vi "String_Conversion_OP110.vi"(11 "String in":string) -> (2 "Array":string[](array[string]), 3 "String out":string)   [LabVIEW 2017]
panel:
  out "spreadsheet string":string
  out "array":string[](array[string])
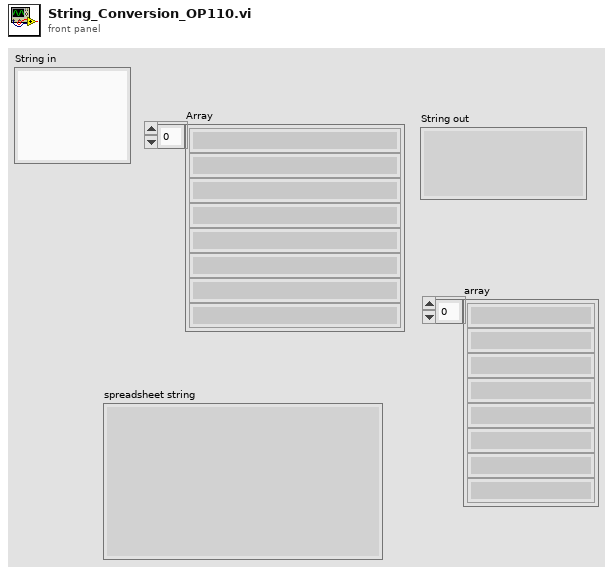
[diagram p1: front panel]
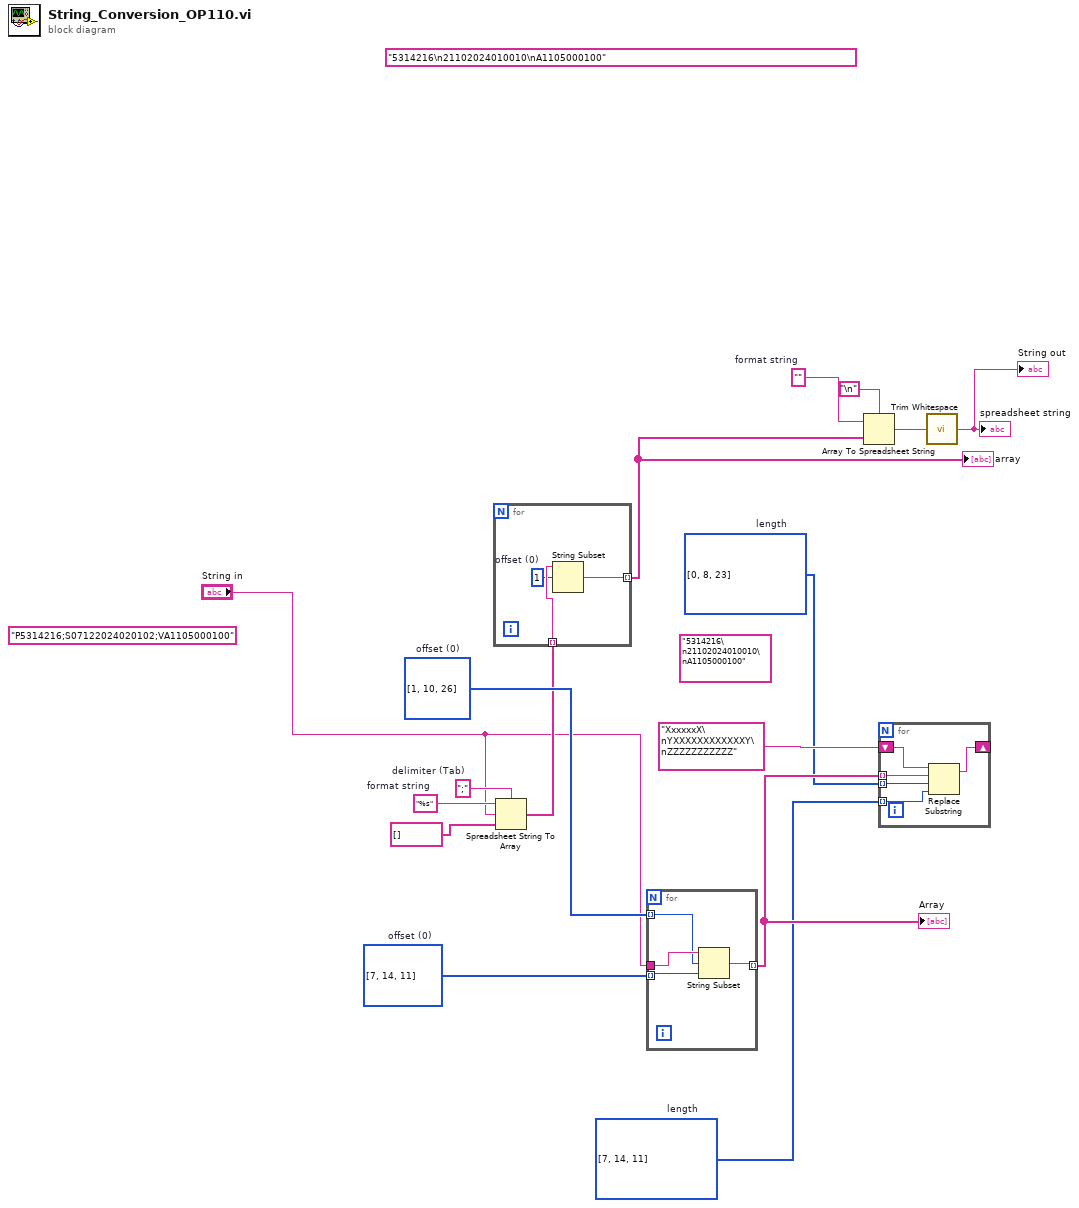
[diagram p0: block diagram]
diagram:
  w5 = ""  # format string
  (unwired) "5314216\n21102024010010\nA1105000100"
  w8 = ";"  # delimiter (Tab)
  w10 = "%s"  # format string
  w11 = i32[] [0, 8, 23]  # length
  (unwired) "5314216\n21102024010010\nA1105000100"
  (unwired) "P5314216;S07122024020102;VA1105000100"
  w14 = i32[] [7, 14, 11]  # length
  w13 = i32[] [7, 14, 11]  # offset (0)
  w12 = i32[] [1, 10, 26]  # offset (0)
  n1 = Spreadsheet String To Array(delimiter (Tab)=w8, format string=w10, spreadsheet string="String in", array type (2D Dbl)=string[] []) -> (array=w7:string[])
  n2 = for {
    tunnel: w7 -> [w19] mode=indexing
    tunnel: [w17] -> w6 mode=indexing
    w18 = 1  # offset (0)
    n3 = String Subset(string=w19, offset (0)=w18) -> (substring=w17:string)  [unwired: 1 in]
  }
  "array" <- w6
  n4 = for {
    tunnel: w12 -> [w22] mode=indexing
    tunnel: w13 -> [w21] mode=indexing
    tunnel: "String in" -> [w23]
    tunnel: [w20] -> w16 mode=indexing
    n5 = String Subset(string=w23, offset (0)=w22, length (rest)=w21) -> (substring=w20:string)
  }
  "Array" <- w16
  n6 = Array To Spreadsheet String(delimiter (Tab)="\n", array=w6, 3:w5) -> (spreadsheet string=w3:string)
  n7 = for {
    tunnel: w14 -> [w28] mode=indexing
    shift-right: [w27] -> _
    shift-left: "XxxxxxX\nYXXXXXXXXXXXXY\nZZZZZZZZZZZ" -> [w26]
    tunnel: w16 -> [w25] mode=indexing
    tunnel: w11 -> [w24] mode=indexing
    n8 = Replace Substring(2:w28, 3:w24, 4:w25, 5:w26) -> (1:w27:string)  [unwired: 1 out]
  }
  n9 = call <vilib>:"Trim Whitespace.vi"("string"=w3) -> ("trimmed string"=→"String out" →"spreadsheet string":string)  [unwired: 1 in]
